vi "CRYFlatten Data Save.vi"(6 "error in":errorcluster, 8 "Any Flatten Data":string, 9 "Path In":path) -> (0 "error out":errorcluster, 3 "Path Out":path)   [LabVIEW 2013]
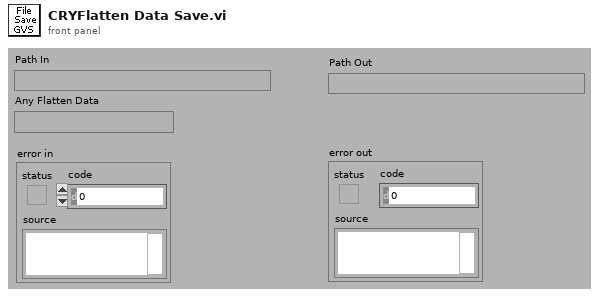
[diagram p1: front panel]
types:
  T1 = enum16{"open", "replace", "create", "open or create", "replace or create", "replace or create with confirmation"}
  T2 = enum16{"big-endian, network order", "native, host order", "little-endian"}
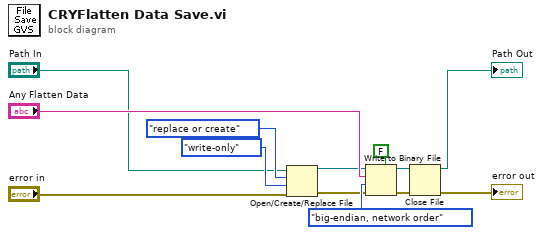
[diagram p0: block diagram]
diagram:
  n1 = Open/Create/Replace File(file path (use dialog)="Path In", error in="error in", operation (0:open)=T1."replace or create", access (0:read/write)=enum16{"read/write", "read-only", "write-only"}."write-only") -> (refnum out=w8:refnum<file>, error out=w5:errorcluster)  [unwired: 3 out]
  n2 = Write to Binary File(file (use dialog)=w8, data="Any Flatten Data", error in=w5, 5:FALSE ("prepend array or string size? (T)"), 9:T2."big-endian, network order" ("Byte Order")) -> (refnum out=w7:refnum<file>, error out=w6:errorcluster)  [unwired: 2 out]
  n3 = Close File(refnum=w7, error in=w6) -> (path=→"Path Out":path, error out=→"error out":errorcluster)
